vi "Validate Single Resource.vi"(8 "error in (no error)":errorcluster, 10 "resources":T1[](array[typedef])) -> (0 "error out":errorcluster, 2 "resource":T1)   [LabVIEW 2020, in "MeasurementLink Pin Map.lvlib"]
uses:
  MeasurementLink Pin Map.lvlib
  MeasurementLink Measurement Server/Helpers/Error Strings Global Internal.vi
  MeasurementLink Pin Map Client/RPC Messages/ni_measurementlink_pinmap_v1_ChannelMapping.ctl
  MeasurementLink Pin Map Client/MeasurementLink Pin Map Client.lvlib
  MeasurementLink Pin Map Client/RPC Messages/ni_measurementlink_pinmap_v1_ResourceAccessInformation.ctl
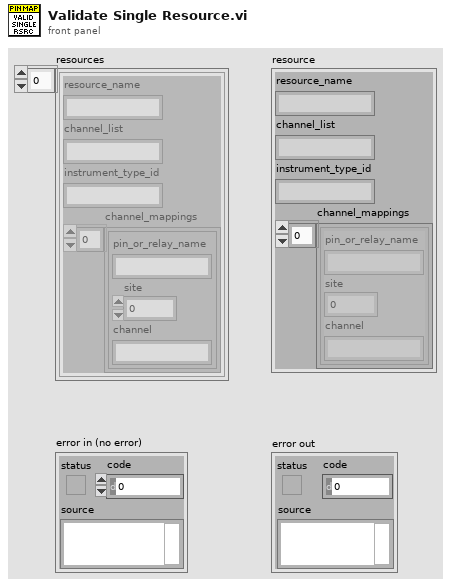
[diagram p1: front panel]
types:
  T1 = typedef "MeasurementLink Pin Map Client.lvlib/ni_measurementlink_pinmap_v1_ResourceAccessInformation.ctl" = cluster{"resource_name":string, "channel_list":string, "instrument_type_id":string, "channel_mappings":T2[]}
  T2 = typedef "MeasurementLink Pin Map Client.lvlib/ni_measurementlink_pinmap_v1_ChannelMapping.ctl" = cluster{"pin_or_relay_name":string, "site":i32, "channel":string}
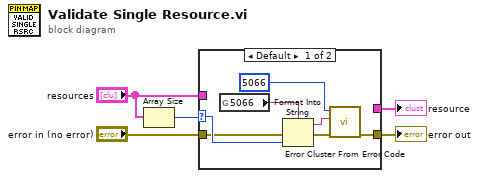
[diagram p0: block diagram]
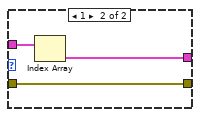
[diagram p2: hidden frame]
diagram:
  n1 = Array Size(array="resources") -> (size(s)=w5:i32)
  n2 = case shown="Default" w5 {
    selector: w5 -> [w8 _]
    tunnel: "resources" -> [_ w15]
    tunnel: [_ w14] -> w3
    tunnel: "error in (no error)" -> [w7 w13]
    tunnel: [w10 w13] -> w1
    frame Default {
      n3 = global read "Error Strings Global Internal.vi" "5066"() -> (w9:string)
      n4 = Format Into String(format string=w9, error in=w7, w8) -> (resulting string=w11:string, error out=w6:errorcluster)  [unwired: 1 in]
      n5 = call <vilib>:"Error Cluster From Error Code.vi"("error in (no error)"=w6, "error message (\"\")"=w11, "error code (0)"=5066) -> ("error out"=w10:errorcluster)  [unwired: 6 in]
    }
    frame 1 {
      n6 = Index Array(array=w15) -> (element=w14:T1)  [unwired: 1 in]
    }
  }
  "resource" <- w3
  "error out" <- w1
